vi "calculate_imsubtraction_value.vi"(9 "Input \nparameters":T2={"Frame rate (ms)"=2000, "Worm strain"="N2", "# Images"=0, "State"=enum."Image acquisition", "Time elapsed"=0.0, "Max_num_runs"=100000, "#TTL"=0, "Time of start TTL"=100000, "ImSub Value"=0, "Time of last TTL"=0, "Number of Columns"=2, "Number of Rows"=2, "# AdjacentTTL"=0, "Sleep deprivation status"="", "Sleep Detection"=FALSE, "# Sleep detections"=0, "Time of first sleep detection"=0, "Time max # adjacent TTL"=0, "Image t-1"=[], "Image t"=[]} {"Number of Rows" items=["1"=1, "2"=2, "3"=3, "4"=4]; "Number of Columns" items=["1"=1, "2"=2, "3"=3, "4"=4]}) -> (1 "Output \nparameters":T2={"Frame rate (ms)"=2000, "Worm strain"="N2", "# Images"=0, "State"=enum."Image acquisition", "Time elapsed"=0.0, "Max_num_runs"=100000, "#TTL"=0, "Time of start TTL"=100000, "ImSub Value"=0, "Time of last TTL"=0, "Number of Columns"=2, "Number of Rows"=2, "# AdjacentTTL"=0, "Sleep deprivation status"="", "Sleep Detection"=FALSE, "# Sleep detections"=0, "Time of first sleep detection"=0, "Time max # adjacent TTL"=0, "Image t-1"=[], "Image t"=[]} {"Number of Rows" items=["1"=1, "2"=2, "3"=3, "4"=4]; "Number of Columns" items=["1"=1, "2"=2, "3"=3, "4"=4]}, 2 "Image subtraction\nvalue":i32)   [LabVIEW 2011]
uses:
  state.ctl
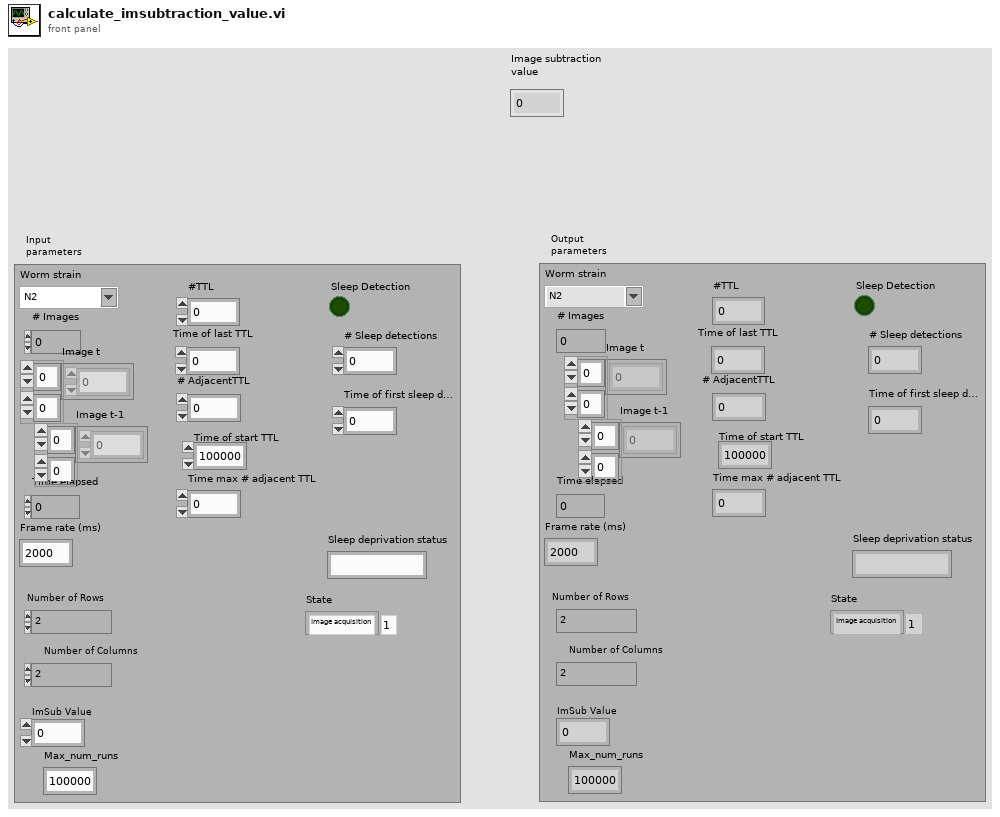
[diagram p1: front panel]
types:
  T1 = typedef "state.ctl" = enum16{"Initialize measurement", "Image acquisition", "Image processing", "Sleep detection", "Control TTL protocol ", "Sleep deprivation", "Update image & exit condition", "Wait "}
  T2 = cluster{"Frame rate (ms)":u32, "Worm strain":string, "# Images":i32, "State":T1, "Time elapsed":dbl, "Max_num_runs":i32, "#TTL":i32, "Time of start TTL":i32, "ImSub Value":i32, "Time of last TTL":i32, "Number of Columns":u32, "Number of Rows":u32, "# AdjacentTTL":i32, "Sleep deprivation status":string, "Sleep Detection":bool, "# Sleep detections":i32, "Time of first sleep detection":i32, "Time max # adjacent TTL":i32, "Image t-1":i32[][], "Image t":i32[][]}
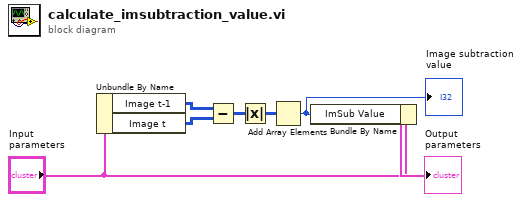
[diagram p0: block diagram]
diagram:
  n1 = Unbundle By Name("Input \nparameters") -> ("Image t-1"=w4:i32[][], "Image t"=w3:i32[][])
  n2 = Subtract ("Subtract.vi")(x=w4, y=w3) -> (x-y=w7:i32[][])
  n3 = Absolute Value ("Absolute Value.vi")(x=w7) -> (abs(x)=w6:i32[][])
  n4 = Add Array Elements(numeric array=w6) -> (sum=w1:i32)
  "Image subtraction\nvalue" <- w1
  n5 = Bundle By Name(cluster="Input \nparameters", "ImSub Value"=w1) -> (→"Output \nparameters":T2)
